vi "Handle Request.vi"(7 "Processing In":refnum<class "Processing.lvclass">, 11 "TestQueryAuth in":refnum<class "TestQueryAuth.lvclass">) -> (0 "error out":errorcluster, 5 "Processing":refnum<class "Processing.lvclass">)   [LabVIEW 2020, in "TestQueryAuth.lvclass"]
uses:
  TestQueryAuth.lvclass
  TestQueryAuth.lvclass/TestQueryAuth.ctl
  <vilib>/IlluminatedG/lv-stream/URI/URI.lvclass
  <vilib>/IlluminatedG/IG HTTP Utils/HTTP Utils/Request/Request.lvclass
  <vilib>/IlluminatedG/IG HTTP Server/HTTP Server/Processing/Processing.lvclass
  <vilib>/IlluminatedG/IG HTTP Utils/HTTP Utils/Redirect Response/Redirect Response.lvclass
  C:/Program Files (x86)/National Instruments/LabVIEW 2020/vi.lib/IlluminatedG/IG HTTP Utils/HTTP Utils/Response/Response.lvclass
  C:/Program Files (x86)/National Instruments/LabVIEW 2020/vi.lib/IlluminatedG/IG HTTP Utils/HTTP Utils/Redirect Response/Redirect Response.lvclass
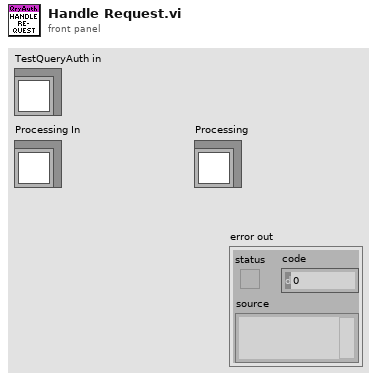
[diagram p1: front panel]
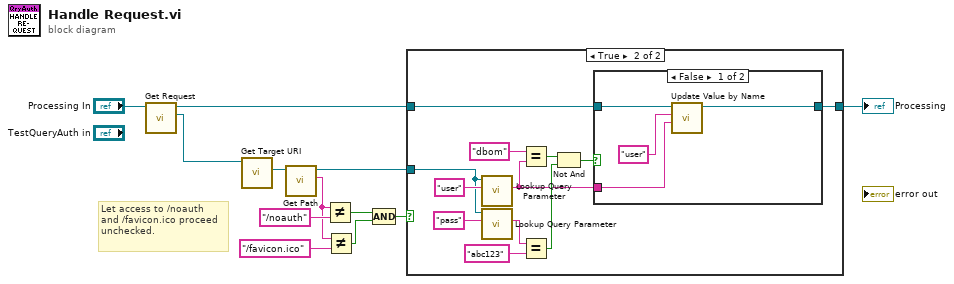
[diagram p0: block diagram]
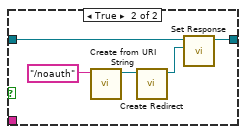
[diagram p3: hidden frame]
diagram:
  # "Let access to /noauth and /favicon.ico proceed unchecked."
  n1 = call <vilib>:"Get Request.vi"("Processing in"="Processing In") -> ("Request"=w4:refnum<class "Request.lvclass">, "Processing out"=w2:refnum<class "Processing.lvclass">)  [unwired: 9 in]
  n2 = call <vilib>:"Get Target URI.vi"("Request in"=w4) -> ("Target URI"=w12:refnum<class "URI.lvclass">)  [unwired: 8 in, 2 out]
  n3 = call <vilib>:"Get Path.vi"("URI in"=w12) -> ("Path"=w8:string, "URI out"=w10:refnum<class "URI.lvclass">)  [unwired: 8 in, 1 out]
  n4 = Not Equal?(x=w8, y="/noauth") -> (x != y?=w7:bool)
  n5 = Not Equal?(x=w8, y="/favicon.ico") -> (x != y?=w6:bool)
  n6 = Compound Arithmetic op=AND(w7, w6) -> (w5:bool)
  n7 = case shown="True" w5 {
    tunnel: w10 -> [_ w16]
    tunnel: w2 -> [w13 w15]
    tunnel: [w13 w14] -> w1
    frame False {
    }
    frame True {
      n8 = call <vilib>:"Lookup Query Parameter.vi"("Name"="user", "URI in"=w16) -> ("Value"=w17:string)  [unwired: 6 in, 3 out]
      n9 = call <vilib>:"Lookup Query Parameter.vi"("Name"="pass", "URI in"=w16) -> ("Value"=w23:string)  [unwired: 6 in, 3 out]
      n10 = Equal?(x="dbom" ("y"), y=w17) -> (x = y?=w20:bool)
      n11 = Equal?(x=w23, y="abc123") -> (x = y?=w19:bool)
      n12 = Not And(1:w19, 2:w20) -> (0:w18:bool)
      n13 = case shown="False" w18 {
        tunnel: w17 -> [w29 _]
        tunnel: w15 -> [w27 w33]
        tunnel: [w26 w32] -> w14
        frame False {
          n14 = call <vilib>:"Update Value by Name.vi"("Value"=w29, "Name"="user", "Processing in"=w27) -> ("Processing out"=w26:refnum<class "Processing.lvclass">)  [unwired: 7 in, 1 out]
        }
        frame True {
          n15 = call <vilib>:"Create from URI String.vi"("URI String"="/noauth") -> ("URI out"=w31:refnum<class "URI.lvclass">)  [unwired: 9 in, 1 out]
          n16 = call <vilib>:"Create Redirect.vi"("Redirect URI"=w31) -> ("Redirect Response out"=w30:refnum<class "Redirect Response.lvclass">)  [unwired: 9 in, 1 out]
          n17 = call <vilib>:"Set Response.vi"("Response"=w30, "Processing in"=w33) -> ("Processing out"=w32:refnum<class "Processing.lvclass">)  [unwired: 9 in]
        }
      }
    }
  }
  "Processing" <- w1
